vi "未命名 6.vi"() -> ()   [LabVIEW 2018]
panel:
  out "波形图 2":cluster{i32, i32, dbl[][]}(graph)
  out "波形图":cluster{i32, i32, dbl[][]}(graph)
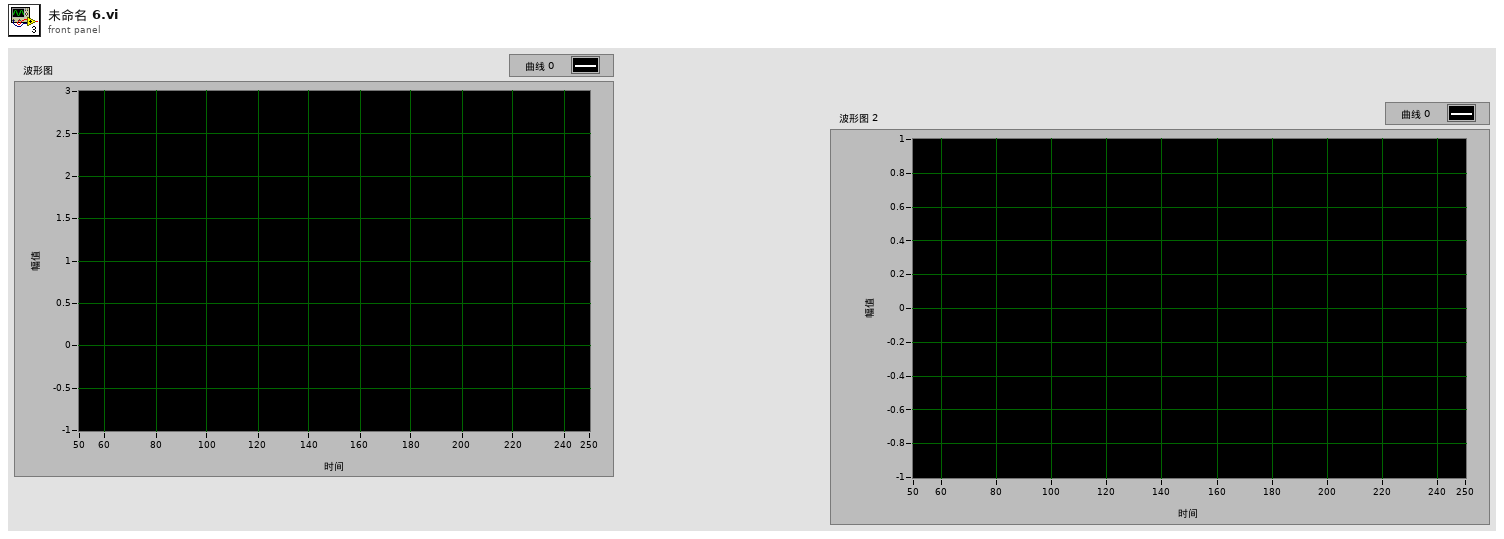
[diagram p1: front panel]
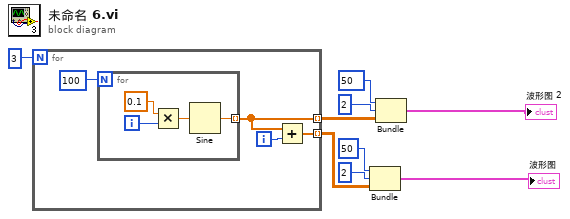
[diagram p0: block diagram]
diagram:
  n1 = for {
    N: 3 -> [_]
    tunnel: [w11] -> w8 mode=indexing
    tunnel: [w10] -> w6 mode=indexing
    i -> [w12]
    n2 = for {
      N: 100 -> [_]
      tunnel: [w14] -> w11 mode=indexing
      i -> [w17]
      n3 = Multiply(x=0.1, y=w17) -> (x*y=w15:dbl)
      n4 = Sine(x=w15) -> (sin(x)=w14:dbl)
    }
    n5 = Add(x=w11, y=w12) -> (x+y=w10:dbl[])
  }
  n6 = Bundle(50, 2, w6) -> (→"波形图":cluster{i32, i32, dbl[][]})  [unwired: 1 in]
  n7 = Bundle(50, 2, w8) -> (→"波形图 2":cluster{i32, i32, dbl[][]})  [unwired: 1 in]
